vi "Get ParentRef Until Type Matched.vi"(5 "Class Name":string, 6 "Error in":errorcluster caption="Error in (no error)", 9 "reference in":refnum<vi>) -> (0 "Error out":errorcluster, 3 "Target Ref":refnum<vi>)   [LabVIEW 2017, in "CSM-Helper.lvclass"]
doc: "-- <b>Controls</b> --\n- <b>Class Name</b>:\n- <b>reference in</b>:\n\n-- <b>Indicators</b> --\n- <b>Target Ref</b>:"
uses:
  CSM-Helper.lvclass
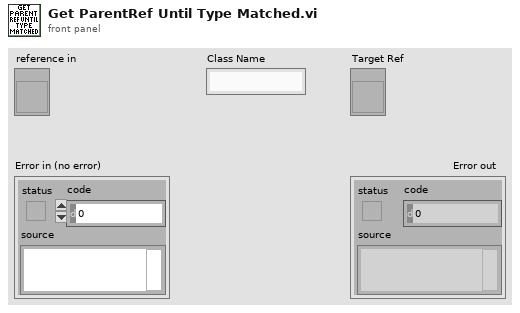
[diagram p1: front panel]
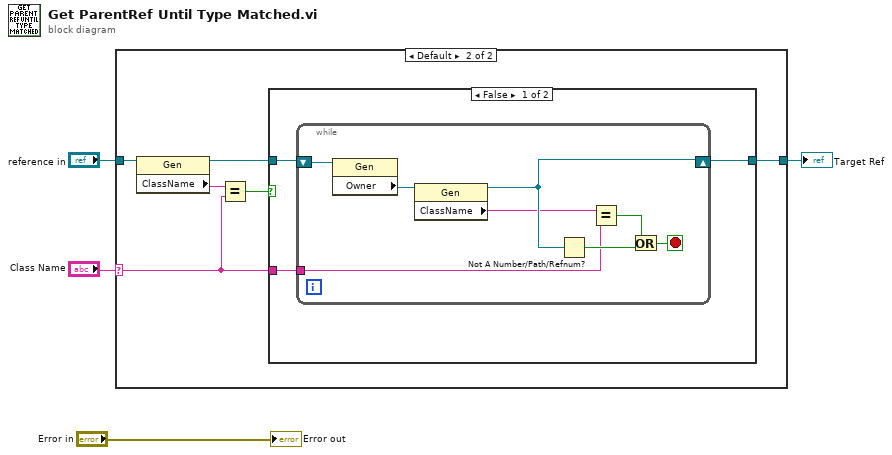
[diagram p0: block diagram]
diagram:
  n1 = case shown="Default" "Class Name" {
    selector: "Class Name" -> [_ w6]
    tunnel: [_ w10] -> w4
    tunnel: "reference in" -> [_ w9]
    frame "" {
    }
    frame Default {
      n2 = property class="Gen"(reference=w9) -> (reference out=w8:refnum<vi>, "ClassName"=w7:string)  [unwired: 1 in, 1 out]
      n3 = Equal?(x=w7, y=w6) -> (x = y?=w5:bool)
      n4 = case shown="False" w5 {
        tunnel: [w13 w22] -> w10
        tunnel: w8 -> [w12 w22]
        tunnel: w6 -> [w11 _]
        frame False {
          n5 = while {
            tunnel: w11 -> [w16]
            shift-right: [w15] -> w13
            shift-left: w12 -> [w21]
            stop <- w20 stop-if-true
            n6 = property class="Gen"(reference=w21) -> ("Owner"=w17:refnum<vi>)  [unwired: 1 in, 2 out]
            n7 = property class="Gen"(reference=w17) -> (reference out=w15:refnum<vi>, "ClassName"=w14:string)  [unwired: 1 in, 1 out]
            n8 = Not A Number/Path/Refnum?(number/path/refnum=w15) -> (NaN/Path/Refnum?=w19:bool)
            n9 = Equal?(x=w14, y=w16) -> (x = y?=w18:bool)
            n10 = Or(x=w18, y=w19) -> (x .or. y?=w20:bool)
          }
        }
        frame True {
        }
      }
    }
  }
  "Target Ref" <- w4
  "Error out" <- "Error in"
